vi "OFBS_test_Mahalanobis.vi"(6 "Test Data":T1, 7 "Parameters":i32[](array[numeric]), 8 "error in (no error)":errorcluster, 9 "Mean vectors":dbl[][](array[numeric]), 10 "Covariance matricies (inversed)":dbl[][][](array[numeric]), 11 "OFBS class in":refnum<class "OptFreqBandsSearch.lvclass">) -> (0 "error out":errorcluster, 1 "Confusion Matrix":i32[][](array[numeric]), 2 "Accuracy":dbl, 3 "OFBS class out":refnum<class "OptFreqBandsSearch.lvclass">)   [LabVIEW 2016, in "Optimal Frequency Bands Search.lvlib" / "OptFreqBandsSearch.lvclass"]
doc: "Метод, реализующий тестирование классификатора на основе многослойного персептрона. Для тестирования могут использоваться обучающие, либо тестовые данные"
uses:
  OptFreqBandsSearch.lvclass
  OFBS_DataTypes.ctl
  OptFreqBandsSearch.lvclass/OptFreqBandsSearch.ctl
  <vilib>/Analysis/baseanly.llb/Vector x A.vi
  <vilib>/Analysis/baseanly.llb/Real Dot Product.vi
  4. Accuracy Assessment for EEG Classification/_vlib/CU_CohenKappa.vi
  <vilib>/addons/Machine Learning/NILabs_MLT.lvlib
  <vilib>/Analysis/NI_AALBase.lvlib
  Optimal Frequency Bands Search.lvlib
  4. Accuracy Assessment for EEG Classification/Classifier.lvlib
panel:
  # "This VI is a part of BCI Design library, http://www.ru-bci.org \nCopyright © 2020, Sotnikov Peter, All rights reserved. License: GNU GPLv3"
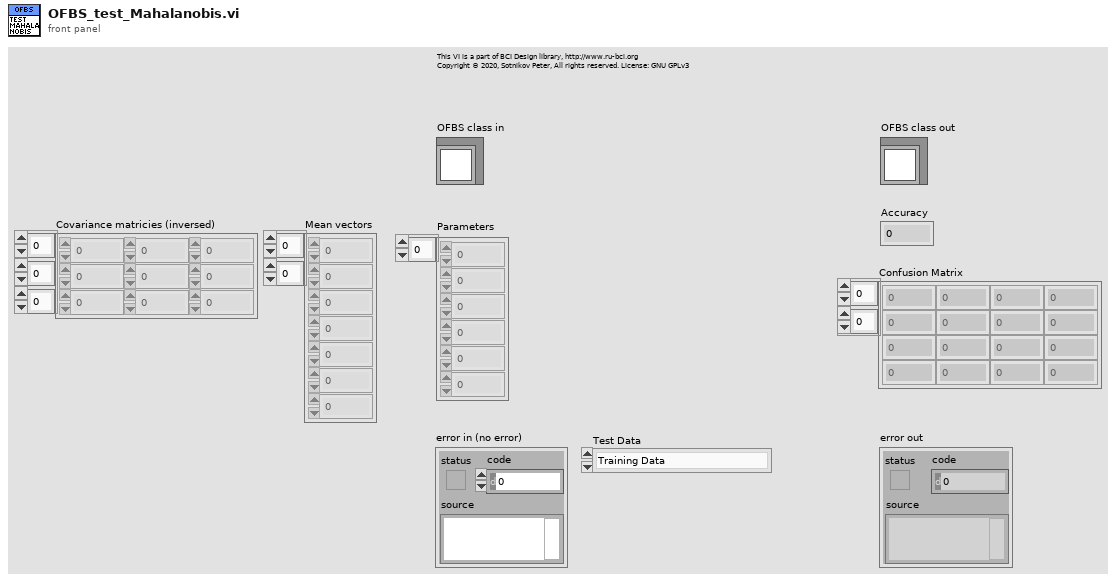
[diagram p1: front panel]
types:
  T1 = typedef "Optimal Frequency Bands Search.lvlib/OFBS_DataTypes.ctl" = enum16{"Training Data", "Test Data", "Training Data (cross-check)", "Test Data (cross-check)"}
  T2 = typedef "Classifier.lvlib/CU_ClassifierQualityMeasure.ctl" = enum16{"Accuracy", "Cohen's kappa"}
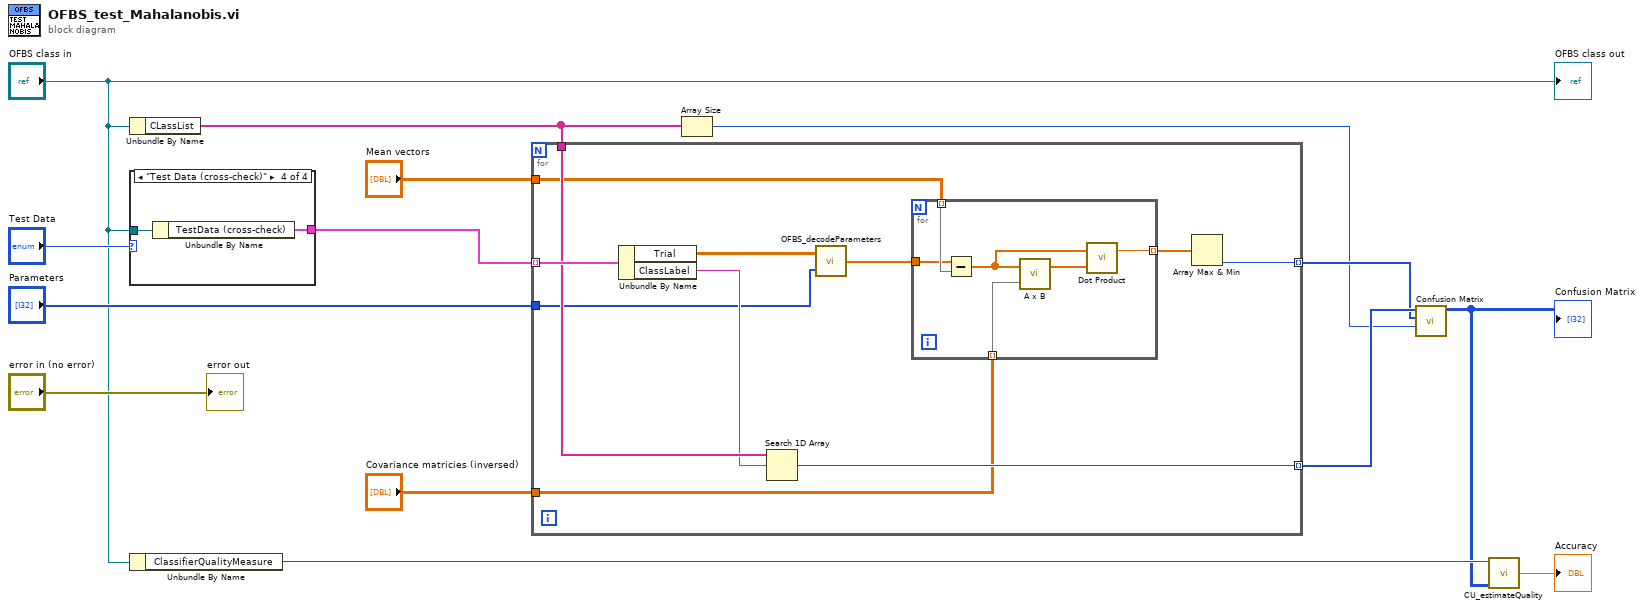
[diagram p0: block diagram]
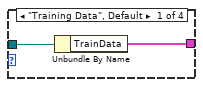
[diagram p2: hidden frame]
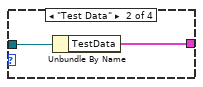
[diagram p3: hidden frame]
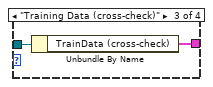
[diagram p4: hidden frame]
diagram:
  n1 = Unbundle By Name("OFBS class in") -> ("CLassList"=w6:string[])
  n2 = case shown="\"Test Data (cross-check)\"" "Test Data" {
    tunnel: "OFBS class in" -> [w16 w18 w20 w22]
    tunnel: [w15 w17 w19 w21] -> w10
    frame "Training Data", Default {
      n3 = Unbundle By Name(w16) -> ("TrainData"=w15:cluster{"ClassLabel":string, "Trial":dbl[][]}[])
    }
    frame "Test Data" {
      n4 = Unbundle By Name(w18) -> ("TestData"=w17:cluster{"ClassLabel":string, "Trial":dbl[][]}[])
    }
    frame "Training Data (cross-check)" {
      n5 = Unbundle By Name(w20) -> ("TrainData (cross-check)"=w19:cluster{"ClassLabel":string, "Trial":dbl[][]}[])
    }
    frame "Test Data (cross-check)" {
      n6 = Unbundle By Name(w22) -> ("TestData (cross-check)"=w21:cluster{"ClassLabel":string, "Trial":dbl[][]}[])
    }
  }
  n7 = Unbundle By Name("OFBS class in") -> ("ClassifierQualityMeasure"=w4:T2)
  n8 = for {
    tunnel: w10 -> [w33] mode=indexing
    tunnel: "Parameters" -> [w24]
    tunnel: w6 -> [w32]
    tunnel: [w30] -> w8 mode=indexing
    tunnel: [w26] -> w7 mode=indexing
    tunnel: "Mean vectors" -> [w29]
    tunnel: "Covariance matricies (inversed)" -> [w28]
    n9 = Unbundle By Name(w33) -> ("Trial"=w25:dbl[][], "ClassLabel"=w31:string)
    n10 = Search 1D Array(1D array=w32, element=w31) -> (index of element=w30:i32)  [unwired: 1 in]
    n11 = call "OFBS_decodeParameters.vi"("Parameters"=w24, "Trial"=w25) -> ("FeatureVector"=w23:dbl[])
    n12 = for {
      tunnel: w29 -> [w39] mode=indexing
      tunnel: w28 -> [w38] mode=indexing
      tunnel: [w35] -> w27 mode=indexing
      tunnel: w23 -> [w34]
      n13 = Subtract(x=w34, y=w39) -> (x-y=w37:dbl[])
      n14 = call-poly <vilib>:"A x B.vi"("Matrix A"=w38, "Vector V'"=w37) -> ("V' x A"=w36:dbl[])  [unwired: 1 out]
      n15 = call-poly <vilib>:"Dot Product.vi"("Y Vector"=w36, "X Vector"=w37) -> ("X * Y"=w35:dbl)  [unwired: 1 out]
    }
    n16 = Array Max & Min(array=w27) -> (min index (indices)=w26:i32)  [unwired: 3 out]
  }
  n17 = Array Size(array=w6) -> (size(s)=w5:i32)
  n18 = call <vilib>:"Confusion Matrix.vi"("# of classes"=w5, "Predicted class labels"=w7, "Actual class labels"=w8) -> ("Confusion Matrix"=w2:i32[][])  [unwired: 7 in, 1 out]
  "Confusion Matrix" <- w2
  n19 = call "CU_estimateQuality.vi"("Quality Measure in"=w4, "Confusion Matrix in"=w2) -> ("Classification Quality out"=→"Accuracy":dbl)  [unwired: 6 in]
  "error out" <- "error in (no error)"
  "OFBS class out" <- "OFBS class in"
